vi "LIN EX Master Write.vi"(5 "CheckType":u8, 6 "DataLen":u8, 7 "pData":string, 9 "PID":u8, 10 "LINIndex":u8, 11 "DevHandle":i32) -> (2 "function return":i32, 3 "pData out":string)   [LabVIEW 2010, in "usb2lin_ex.lvlib"]
doc: "int WINAPI LIN_EX_MasterWrite(int DevHandle,unsigned char LINIndex,unsigned char PID,unsigned char *pData,unsigned char DataLen,unsigned char CheckType);"
uses:
  usb2lin_ex.lvlib
  USB2XXX/trunk/USB2XXX/USB2XXX/vs2010/Release/USB2XXX.dll
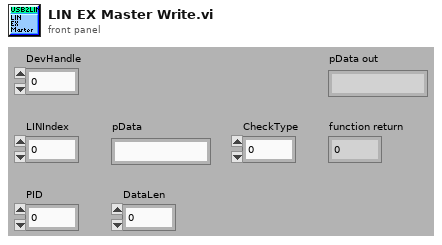
[diagram p1: front panel]
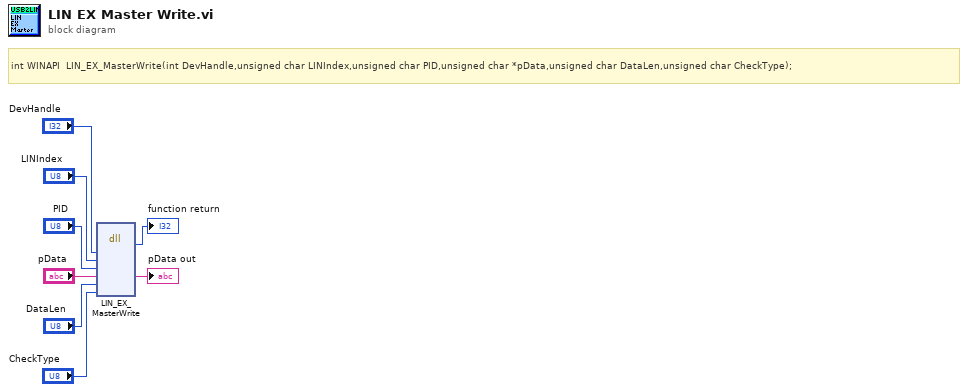
[diagram p0: block diagram]
diagram:
  # "int WINAPI  LIN_EX_MasterWrite(int DevHandle,unsigned char LINIndex,unsigned char PID,unsigned char *pData,unsigned char DataLen,unsigned char CheckType);"
  n1 = dll-call lib="E:/Projects/USB2XXX/trunk/USB2XXX/USB2XXX/vs2010/Release/USB2XXX.*" fn="LIN_EX_MasterWrite"("DevHandle"="DevHandle", "LINIndex"="LINIndex", "PID"="PID", "pData"="pData", "DataLen"="DataLen", "CheckType"="CheckType") -> (→"function return":i32, "pData"=→"pData out":string)  [unwired: 8 in, 2 out]
